vi "Timer Helper Loop.vi"(8 "Timer ID":i32, 9 "Setup Timer":refnum<user-event>, 10 "Stop Helper Loop":refnum<user-event>, 11 "Message Queue":refnum<class "Delacor_lib_QMH_Message Queue.lvclass">) -> ()   [LabVIEW 2015, in "Tool Module.lvlib"]
uses:
  Tool Module.lvlib
  <vilib>/Delacor/Delacor QMH/Libraries/Message Queue_class/Delacor_lib_QMH_Message Queue.lvclass
  Setup Timer Argument--cluster.ctl
  Stop Helper Loop Argument--cluster.ctl
  <vilib>/Delacor/Delacor QMH/Libraries/Message Queue_class/Delacor_lib_QMH_Message Queue.lvclass/Delacor_lib_QMH_Message Queue.ctl
  <vilib>/Delacor/Delacor QMH/Libraries/Message Queue_class/Delacor_lib_QMH_Enqueue Message (Single).vi
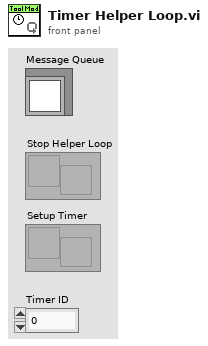
[diagram p1: front panel]
types:
  T1 = cluster{"Period":i32, "Count":i32, "Next State":string, "Enqueue Next State":bool}
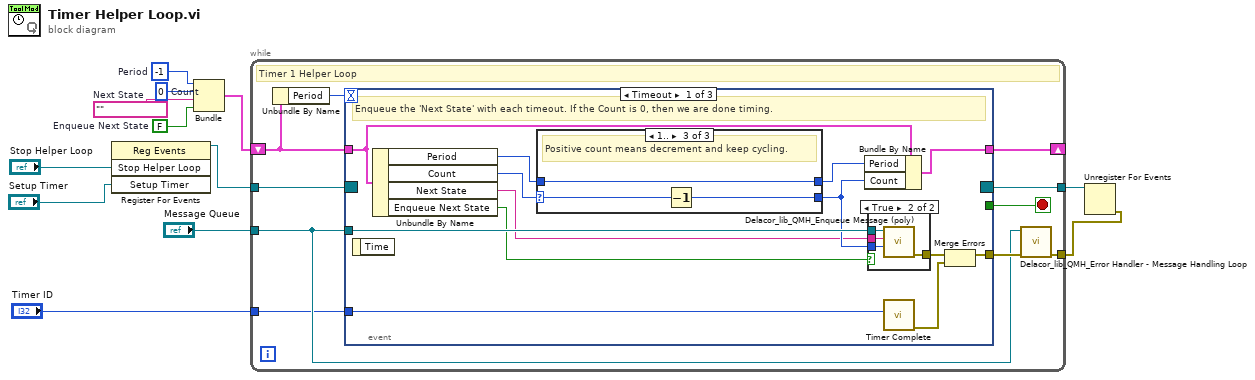
[diagram p0: block diagram]
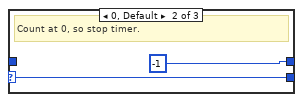
[diagram p4: hidden frame]
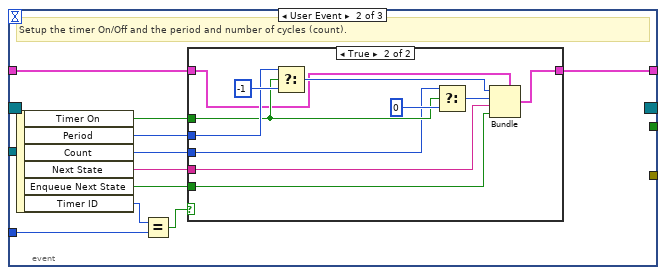
[diagram p5: hidden frame]
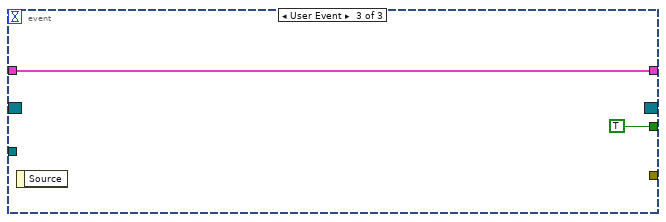
[diagram p7: hidden frame]
diagram:
  w1 = FALSE  # Enqueue Next State
  w10 = ""  # Next State
  w9 = 0  # Count
  w11 = -1  # Period
  n1 = register-events("Stop Helper Loop", "Setup Timer") -> (reference out=w7:refnum<event-registration>)  [unwired: 2 in, 1 out]
  n2 = Bundle("Period"=w11, "Count"=w9, "Next State"=w10, "Enqueue Next State"=w1) -> (w8:T1)  [unwired: 1 in]
  n3 = while {
    tunnel: "Message Queue" -> [w18]
    tunnel: w7 -> [w20]
    shift-right: [w19] -> _
    shift-left: w8 -> [w17]
    tunnel: [w15] -> w3
    tunnel: [w14] -> w4
    tunnel: "Timer ID" -> [w13]
    stop <- w22 stop-if-true
    # "Timer 1 Helper Loop"
    n4 = Unbundle By Name(w17) -> ("Period"=w16:i32)
    n5 = event shown="[0] Timeout" {
      selector: w20 -> [_ _ _]
      dyn-events: [_ _ _] -> w14
      timeout: w16 -> [_ _ _]
      tunnel: [_ _ TRUE] -> w22
      tunnel: [w27 _ _] -> w21
      tunnel: w17 -> [w23 w51 w69]
      tunnel: [w28 w52 w69] -> w19
      tunnel: w18 -> [w35 _ _]
      tunnel: w13 -> [w25 w50 _]
      event Timeout {
        # "Enqueue the 'Next State' with each timeout. If the Count is 0, then we are done timing."
        n6 = event-data() -> ()  [unwired: 1 in, 1 out]
        n7 = Unbundle By Name(w23) -> ("Period"=w33:i32, "Count"=w32:i32, "Next State"=w29:string, "Enqueue Next State"=w24:bool)
        n8 = case shown="1.." w32 {
          selector: w32 -> [w40 w42 w46]
          tunnel: w33 -> [w41 _ w44]
          tunnel: [w41 -1 ("Period") w44] -> w31
          tunnel: [w40 w42 w45] -> w30
          frame -1 {
            # "-1 means run forever."
          }
          frame 0, Default {
            # "Count at 0, so stop timer."
          }
          frame 1.. {
            # "Positive count means decrement and keep cycling."
            n9 = Decrement(x=w46) -> (x-1=w45:i32)
          }
        }
        n10 = Bundle By Name(cluster=w23, "Period"=w31, "Count"=w30) -> (w28:T1)
        n11 = case shown="True" w24 {
          tunnel: w35 -> [_ w39]
          tunnel: [_ w38] -> w34
          tunnel: w30 -> [_ w37]
          tunnel: w29 -> [_ w36]
          frame False {
          }
          frame True {
            n12 = call-poly <vilib>:"Delacor_lib_QMH_Enqueue Message (poly).vi"("Message Data"=w37, "Message"=w36, "Message Queue in"=w39) -> ("error out"=w38:errorcluster)  [unwired: 7 in, 1 out]
          }
        }
        n13 = call "Timer Complete.vi"("Timer ID"=w25) -> ("error out"=w26:errorcluster)  [unwired: 10 in]
        n14 = Merge Errors(w34, w26) -> (w27:errorcluster)
      }
      event User Event {
        # "Setup the timer On/Off and the period and number of cycles (count)."
        n15 = event-data() -> ("Timer On"=w55:bool, "Period"=w56:i32, "Count"=w54:i32, "Next State"=w53:string, "Enqueue Next State"=w47:bool, "Timer ID"=w48:i32)  [unwired: 1 in]
        n16 = Equal?(x=w48, y=w50) -> (x = y?=w49:bool)
        n17 = case shown="True" w49 {
          tunnel: w56 -> [_ w66]
          tunnel: w55 -> [_ w65]
          tunnel: w54 -> [_ w64]
          tunnel: w53 -> [_ w61]
          tunnel: [w57 w60] -> w52
          tunnel: w51 -> [w57 w59]
          tunnel: w47 -> [_ w58]
          frame False {
          }
          frame True {
            n18 = Select(t=w66, s=w65, f=-1) -> (s? t:f=w63:i32)
            n19 = Select(t=w64, s=w65, f=0) -> (s? t:f=w62:i32)
            n20 = Bundle(cluster=w59, "Period"=w63, "Count"=w62, "Next State"=w61, "Enqueue Next State"=w58) -> (w60:T1)
          }
        }
      }
      event User Event {
        n21 = event-data() -> ()  [unwired: 1 in, 1 out]
      }
    }
    n22 = call-dynamic "Delacor_lib_QMH_Error Handler - Message Handling Loop.vi"("error in (no error)"=w21, "Message Queue in"=w18) -> ("dup error in"=w15:errorcluster)  [unwired: 8 in, 1 out]
  }
  n23 = Unregister For Events(event registration refnum=w4, error in=w3) -> ()  [unwired: 1 out]
